vi "AMC Send Message.vi"(4 "Acknowledge Message (F)":bool, 5 "Receiver Host":string, 6 "Source Process":string, 7 "Receiver Process":string, 8 "error in (no error)":errorcluster, 9 "Priority Message (F)":bool, 10 "Message":T1, 11 "Message Queue in":T3) -> (0 "error out":errorcluster, 3 "Message Queue out":T3)   [LabVIEW 2011, in "ART2 Test Panel.lvlib" / "TLB_Dependencies.lvlib"]
doc: "This VI adds a message to\n- the local queue passed in by reference if the receiver host and process are left undefined\n- another message queue on the local target if the receiver host is undefined, but the receiver process is specified\n- the message dispatch queue to pass the message to another target through the message dispatcher if the receiver host and process are specified."
uses:
  TLB_Dependencies.lvlib
  amc_Message Queue.ctl
  amc_Message.ctl
  Users/rkidagan/Dropbox/Atheros/ART2/Development/ART2 Test Panel/ART2 Test Panel/Components/Dependencies.llb/Keyed Array.ctl
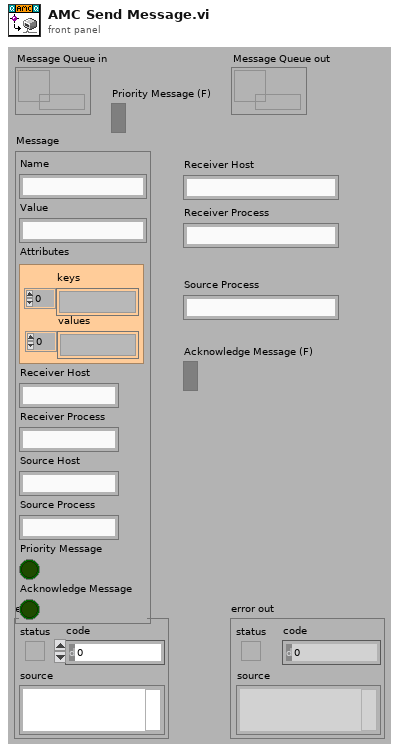
[diagram p1: front panel]
types:
  T1 = typedef "ART2 Test Panel.lvlib/TLB_Dependencies.lvlib/amc_Message.ctl" = cluster{"Name":string, "Value":string, "Attributes":T2, "Receiver Host":string, "Receiver Process":string, "Source Host":string, "Source Process":string, "Priority Message":bool, "Acknowledge Message":bool}
  T2 = typedef "ART2 Test Panel.lvlib/TLB_Dependencies.lvlib/Keyed Array.ctl" = cluster{"keys":string[], "values":string[]}
  T3 = typedef "ART2 Test Panel.lvlib/TLB_Dependencies.lvlib/amc_Message Queue.ctl" = refnum<queue>
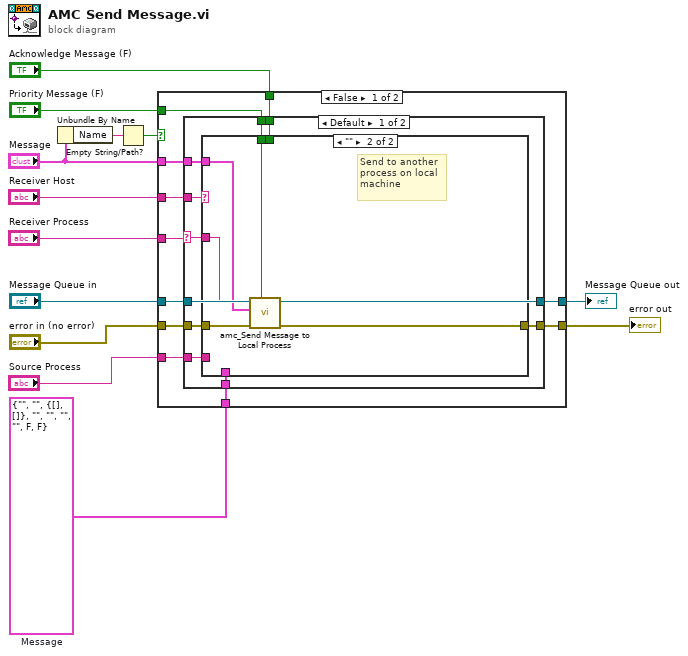
[diagram p0: block diagram]
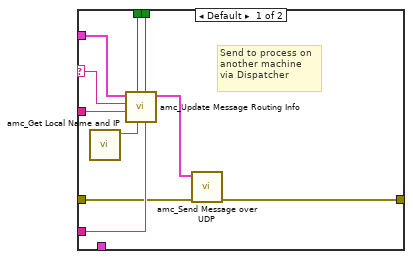
[diagram p2: hidden frame]
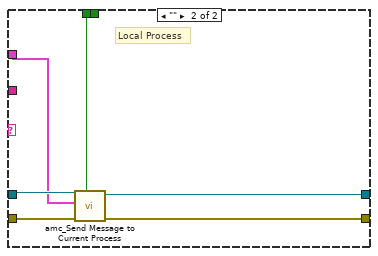
[diagram p3: hidden frame]
diagram:
  w2 = T1 {"Name"="", "Value"="", "Attributes"={"keys"=[], "values"=[]}, "Receiver Host"="", "Receiver Process"="", "Source Host"="", "Source Process"="", "Priority Message"=FALSE, "Acknowledge Message"=FALSE}  # Message
  n1 = Unbundle By Name("Message") -> ("Name"=w7:string)
  n2 = Empty String/Path?(string/path=w7) -> (empty?=w3:bool)
  n3 = case shown="False" w3 {
    tunnel: "error in (no error)" -> [w24 w56]
    tunnel: [w23 w56] -> w12
    tunnel: "Message Queue in" -> [w22 w57]
    tunnel: [w21 w57] -> w10
    tunnel: "Priority Message (F)" -> [w20 _]
    tunnel: "Message" -> [w17 _]
    tunnel: "Receiver Process" -> [w19 _]
    tunnel: "Receiver Host" -> [w18 _]
    tunnel: "Source Process" -> [w16 _]
    tunnel: w2 -> [w15 _]
    tunnel: "Acknowledge Message (F)" -> [w14 _]
    frame False {
      n4 = case shown="Default" w19 {
        selector: w19 -> [w32 _]
        tunnel: w24 -> [w28 w55]
        tunnel: [w30 w54] -> w23
        tunnel: w22 -> [w31 w53]
        tunnel: [w31 w50] -> w21
        tunnel: w20 -> [w33 w52]
        tunnel: w18 -> [w34 _]
        tunnel: w17 -> [w29 w51]
        tunnel: w16 -> [w27 _]
        tunnel: w15 -> [w26 _]
        tunnel: w14 -> [w25 _]
        frame Default {
          n5 = case shown="\"\"" w34 {
            selector: w34 -> [w44 _]
            tunnel: w33 -> [w42 w49]
            tunnel: w32 -> [w39 w47]
            tunnel: [w38 w48] -> w30
            tunnel: w29 -> [w43 w45]
            tunnel: w28 -> [w37 w46]
            tunnel: w27 -> [w41 _]
            tunnel: w26 -> [_ _]
            tunnel: w25 -> [w35 _]
            frame Default {
              # "Send to process on\nanother machine\nvia Dispatcher"
              n6 = call "amc_Get Local Name and IP.vi"() -> ("Name"=w40:string)  [unwired: 1 in, 10 out]
              n7 = call "amc_Update Message Routing Info.vi"("Source Process"=w41, "Acknowledge Message (F)"=w35, "Source Host"=w40, "Priority Message (F)"=w42, "Receiver Process"=w39, "Receiver Host"=w44, "Message"=w43) -> ("Message"=w36:T1)  [unwired: 3 in, 1 out]
              n8 = call "amc_Send Message over UDP.vi"("error in"=w37, "Message"=w36) -> ("error out"=w38:errorcluster)  [unwired: 1 in, 8 out]
            }
            frame "" {
              # "Send to another\nprocess on local\nmachine"
              n9 = call "amc_Send Message to Local Process.vi"("Priority Message (F)"=w49, "error in (no error)"=w46, "Message"=w45, "Process Name"=w47) -> ("error out"=w48:errorcluster)  [unwired: 1 in, 6 out]
            }
          }
        }
        frame "" {
          # "Local Process"
          n10 = call "amc_Send Message to Current Process.vi"("Priority Message (F)"=w52, "error in (no error)"=w55, "Message"=w51, "Message Queue in"=w53) -> ("error out"=w54:errorcluster, "Message Queue out"=w50:T3)  [unwired: 1 in, 5 out]
        }
      }
    }
    frame True {
    }
  }
  "error out" <- w12
  "Message Queue out" <- w10
